vi "Run.vi"(9 "Team In":refnum<class "Team.lvclass">, 11 "MySquare in":refnum<class "MySquare.lvclass">) -> (1 "Team":refnum<class "Team.lvclass">, 2 "Run Result":T1, 3 "MySquare out":refnum<class "MySquare.lvclass">)   [LabVIEW 2020, in "Galaxy.lvlib" / "MySquare.lvclass"]
doc: "This VI is called on every active square each turn of the game for the square to decide what action to take."
uses:
  MySquare.lvclass
  C:/dev/illuminatedg/sol-squarebattle/SquareBattle/Square/Square.lvclass
  SquareBattle/Run Result.ctl
  SquareBattle/Square/Square.lvclass
  SquareBattle/Action.ctl
  SquareBattle/Direction.ctl
  SquareBattle/Team/Team.lvclass
  SquareBattle/Square/Square.lvclass/Square.ctl
  SquareBattle/SquareBattle.lvlib
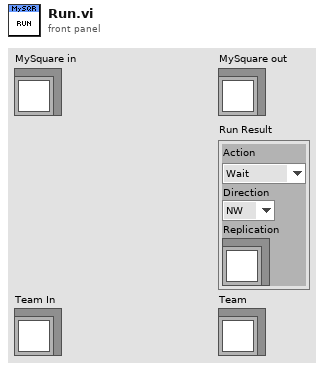
[diagram p1: front panel]
types:
  T1 = typedef "SquareBattle.lvlib/Run Result.ctl" = cluster{"Action":T2, "Direction":T3, "Replication":refnum<class "Square.lvclass">}
  T2 = typedef "SquareBattle.lvlib/Action.ctl" = enum16{"Wait", "Move", "Attack", "Replicate"}
  T3 = typedef "SquareBattle.lvlib/Direction.ctl" = enum16{"NW", "N", "NE", "E", "SE", "S", "SW", "W"}
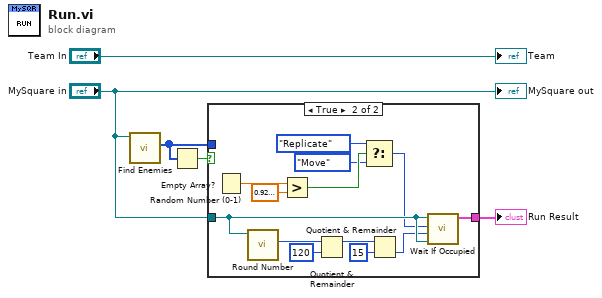
[diagram p0: block diagram]
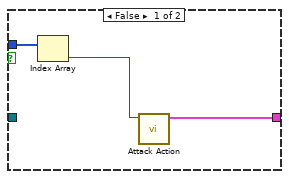
[diagram p2: hidden frame]
diagram:
  n1 = call "Find Enemies.vi"("Square"="MySquare in") -> ("Enemy Directions"=w4:T3[])  [unwired: 10 in]
  n2 = Empty Array?(array=w4) -> (empty?=w5:bool)
  n3 = case shown="True" w5 {
    tunnel: w4 -> [w8 _]
    tunnel: [w6 w11] -> w3
    tunnel: "MySquare in" -> [_ w21]
    frame False {
      n4 = Index Array(array=w8) -> (element=w7:T3)  [unwired: 1 in]
      n5 = call "Attack Action.vi"("Direction"=w7) -> ("Run Result"=w6:T1)  [unwired: 10 in]
    }
    frame True {
      n6 = Random Number (0-1)() -> (number: 0 to 1=w20:dbl)
      n7 = call "Round Number.vi"("Square in"=w21) -> ("Round Number"=w12:u32)  [unwired: 10 in]
      n8 = Greater?(x=w20, y=0.9299999999999999) -> (0:w18:bool)
      n9 = Quotient & Remainder(x=w12, y=120) -> (x-y*floor(x/y)=w13:u32)  [unwired: 1 out]
      n10 = Select(t=Action."Replicate" ("Action"), s=w18, f=Action."Move" ("Action")) -> (s? t:f=w9:T2)
      n11 = Quotient & Remainder(x=w13, y=15) -> (floor(x/y)=w10:u32)  [unwired: 1 out]
      n12 = call "Wait If Occupied.vi"("Replication Square"=w21, "Direction"=w10, "Action if Empty"=w9, "Square In"=w21) -> ("Run Result"=w11:T1)  [unwired: 7 in]
    }
  }
  "Run Result" <- w3
  "MySquare out" <- "MySquare in"
  "Team" <- "Team In"
